vi "Not A Semaphore.vi"(1 "semaphore":T1) -> (0 "not a semaphore":bool)   [LabVIEW 2013]
doc: "Returns TRUE if <B>semaphore</B> is not a valid semaphore refnum."
uses:
  Semaphore Refnum Core.ctl
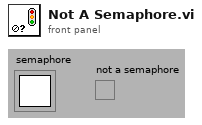
[diagram p1: front panel]
types:
  T1 = typedef "Semaphore RefNum" = refnum<k1>
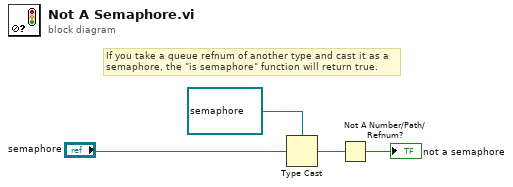
[diagram p0: block diagram]
diagram:
  w3 = refnum<queue> refnum items=["Semaphore Core"] ("queue out")
  # "If you take a queue refnum of another type and cast it as a semaphore, the \"is semaphore\" function will return true."
  n1 = Type Cast(type=w3, x="semaphore") -> (*(type *) &x=w1:refnum<queue>)
  n2 = Not A Number/Path/Refnum?(number/path/refnum=w1) -> (NaN/Path/Refnum?=→"not a semaphore":bool)
